vi "Adjust Control Width.vi"(6 "Control Ref Cluster":T1, 8 "error in (no error)":errorcluster) -> (0 "error out":errorcluster)   [LabVIEW 2017, in "3D Plot.lvclass"]
uses:
  <vilib>/Math Plots/3D Math Plots/3D Plot/3D Plot/3D Plot.lvclass
  <vilib>/Math Plots/3D Math Plots/3D Plot/Action String/3DMathPlot Ctrl Act Cluster.ctl
  <vilib>/Math Plots/3D Math Plots/3D Plot/Action String/3DMathPlot State Class.ctl
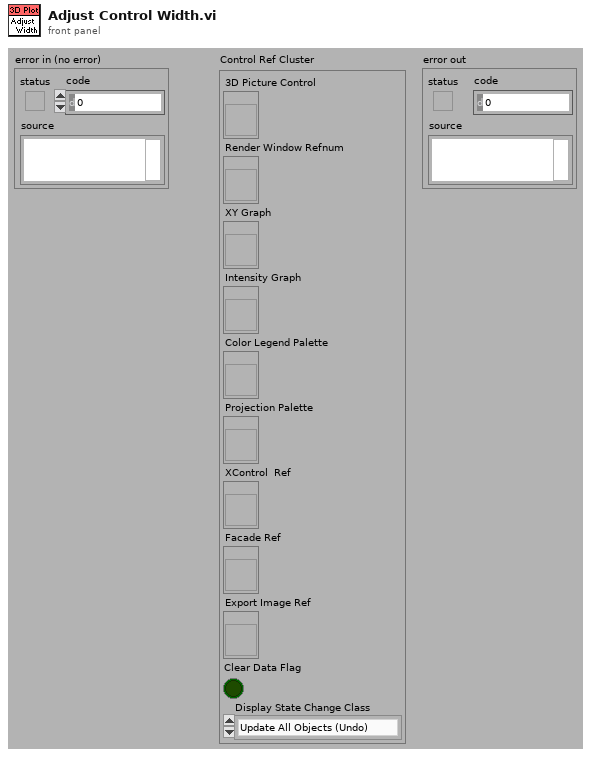
[diagram p1: front panel]
types:
  T1 = typedef "3DMathPlot Ctrl Act Cluster.ctl" = cluster{"3D Picture Control":refnum<vi>, "Render Window Refnum":refnum<vi>, "XY Graph":refnum<vi>, "Intensity Graph":refnum<vi>, "Color Legend Palette":refnum<vi>, "Projection Palette":refnum<vi>, "XControl  Ref":refnum<vi>, "Facade Ref":refnum<vi>, "Export Image Ref":refnum<vi>, "Clear Data Flag":bool, "Display State Change Class":T2}
  T2 = typedef "3DMathPlot State Class.ctl" = enum16{"Update All Objects (Undo)", "Update Light Object Only", "Update Axis Object Only", "Update Plot Object Only", "Update Cursor Object Only", "Update Axis Plot Cursor Objects", "No Update"}
  T3 = enum16{"No Scaling", "Scale All Objects", "Scale Single Object"}
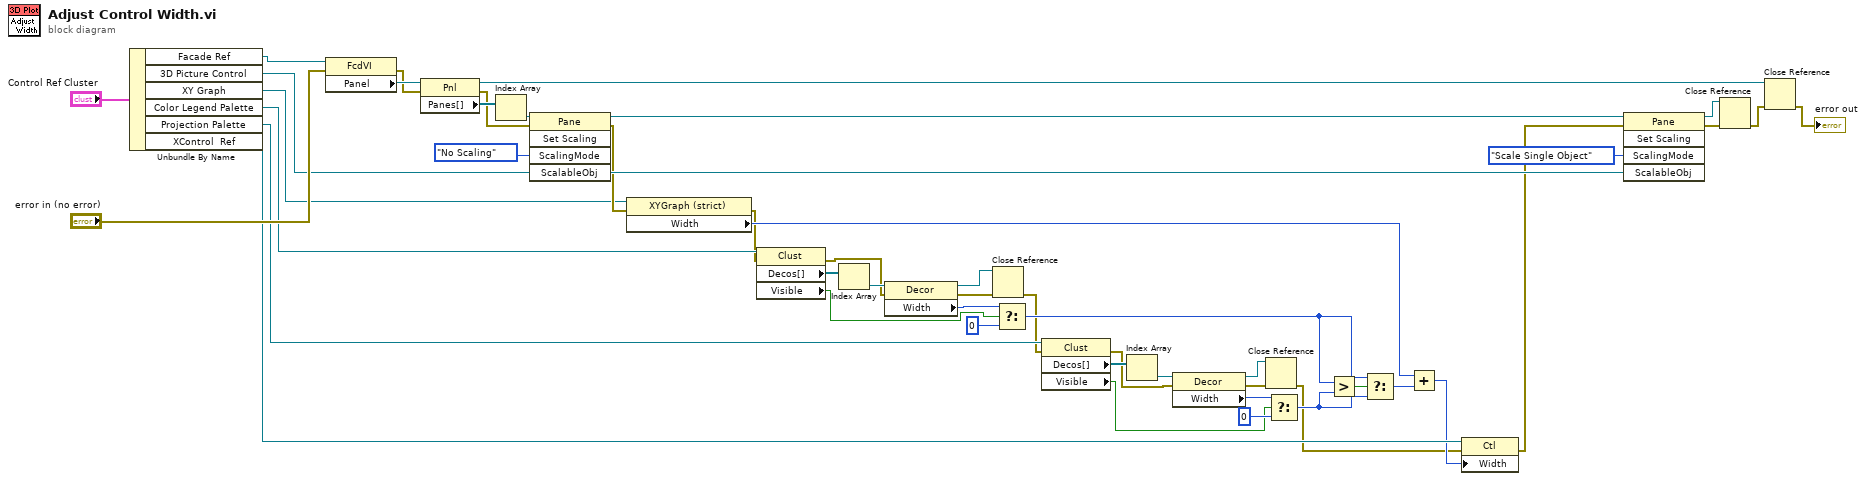
[diagram p0: block diagram]
diagram:
  n1 = Unbundle By Name("Control Ref Cluster") -> ("Facade Ref"=w46:refnum<vi>, "3D Picture Control"=w45:refnum<vi>, "XY Graph"=w22:refnum<vi>, "Color Legend Palette"=w27:refnum<vi>, "Projection Palette"=w26:refnum<vi>, "XControl  Ref"=w23:refnum<vi>)
  n2 = property class="FcdVI"(reference=w46, error in="error in (no error)") -> (error out=w40:errorcluster, "Panel"=w44:refnum<vi>)  [unwired: 1 out]
  n3 = property class="Pnl"(reference=w44, error in=w40) -> (reference out=w11:refnum<vi>, error out=w39:errorcluster, "Panes[]"=w43:refnum<vi>[])
  n4 = Index Array(array=w43) -> (element=w42:refnum<vi>)  [unwired: 1 in]
  n5 = invoke class="Pane" method="Set Scaling"(reference=w42, error in=w39, "ScalingMode"=T3."No Scaling" ("Scaling Mode")) -> (reference out=w38:refnum<vi>, error out=w25:errorcluster)  [unwired: 2 in, 3 out]
  n6 = property class="XYGraph (strict)"(reference=w22, error in=w25) -> (error out=w21:errorcluster, "Width"=w28:u32)  [unwired: 1 out]
  n7 = property class="Clust"(reference=w27, error in=w21) -> (error out=w13:errorcluster, "Decos[]"=w19:refnum<vi>[], "Visible"=w36:bool)  [unwired: 1 out]
  n8 = Index Array(array=w19) -> (element=w18:refnum<vi>)  [unwired: 1 in]
  n9 = property class="Decor"(reference=w18, error in=w13) -> (reference out=w6:refnum<vi>, error out=w4:errorcluster, "Width"=w17:u32)
  n10 = Close Reference(reference=w6, error in (no error)=w4) -> (error out=w3:errorcluster)
  n11 = Select(t=w17, s=w36, f=u32 0) -> (s? t:f=w31:u32)
  n12 = property class="Clust"(reference=w26, error in=w3) -> (error out=w12:errorcluster, "Decos[]"=w15:refnum<vi>[], "Visible"=w33:bool)  [unwired: 1 out]
  n13 = Index Array(array=w15) -> (element=w16:refnum<vi>)  [unwired: 1 in]
  n14 = property class="Decor"(reference=w16, error in=w12) -> (reference out=w5:refnum<vi>, error out=w2:errorcluster, "Width"=w14:u32)
  n15 = Close Reference(reference=w5, error in (no error)=w2) -> (error out=w1:errorcluster)
  n16 = Select(t=w14, s=w33, f=u32 0) -> (s? t:f=w30:u32)
  n17 = Greater?(x=w31, y=w30) -> (0:w32:bool)
  n18 = Select(t=w31, s=w32, f=w30) -> (s? t:f=w29:u32)
  n19 = Add(x=w28, y=w29) -> (x+y=w20:u32)
  n20 = property class="Ctl"(reference=w23, error in=w1, "Width"=w20) -> (error out=w24:errorcluster)  [unwired: 1 out]
  n21 = invoke class="Pane" method="Set Scaling"(reference=w38, error in=w24, "ScalingMode"=T3."Scale Single Object" ("Scaling Mode"), "ScalableObj"=w45) -> (reference out=w10:refnum<vi>, error out=w9:errorcluster)  [unwired: 1 in, 3 out]
  n22 = Close Reference(reference=w10, error in (no error)=w9) -> (error out=w8:errorcluster)
  n23 = Close Reference(reference=w11, error in (no error)=w8) -> (error out=→"error out":errorcluster)
